vi "Meandr_FIFO_target.vi"() -> ()   [LabVIEW 2018]
uses:
  <vilib>/Platform/TimedLoop/XDataNode/timing_clust.ctl
  <vilib>/Platform/TimedLoop/XDataNode/nitl_modes.ctl
  <vilib>/Platform/TimedLoop/XDataNode/wakeup.ctl
  <vilib>/rvi/Emulation/niFpgaGetClockAttributes.vi
  <vilib>/rvi/Emulation/niFpgaSctlEmulationGetInTimedLoop.vi
  <vilib>/rvi/Emulation/niFpgaEmulationReportErrorSimple.vi
  <vilib>/rvi/eio/common/nirviEmuTemplateMethod_errors.vi
  <vilib>/rvi/Emulation/niFpgaCriticalErrorInLSC.vi
  <vilib>/rvi/Emulation/niFpgaProcessEmulError.vi
  <vilib>/rvi/interface/RandomDataEmulation/niFpgaRandomDataHandleErrors.vi
  <vilib>/eio/EIONode/EIONode.xnode
  <vilib>/Platform/TimedLoop/XDataNode/XDataNode.xnode
  <vilib>/rvi/DataTransferAndStorage/Container/XNode/niFpgaContainer.xnode
  <vilib>/rvi/interface/RandomDataEmulation/nirviRandomDataFpgaReadWriteTemplate.vi
  <vilib>/Platform/TimedLoop/XDataNode/XDNodeRunTimeDep.lvlib
panel:
  in  "stop 2":bool
  in  "Push?":bool
  in  "Source Freq":refnum<k21>="100 MHz Clock"
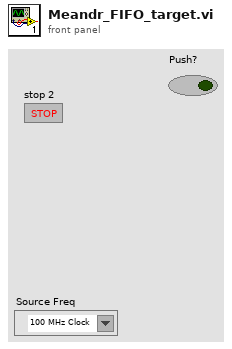
[diagram p1: front panel]
types:
  T1 = typedef "XDNodeRunTimeDep.lvlib/timing_clust.ctl" = cluster{"Expected End [f-1]":u64, "Actual End [f-1]":u64, "Finished Late? [f-1]":bool, "Expected End [i-1]":u64, "Actual End [i-1]":u64, "Finished Late? [i-1]":bool, "Expected Start [i]":u64, "Actual Start [i]":u64, "Expected Start [f]":u64, "Actual Start [f]":u64, "Source Name":string, "Structure Name":string, "Period":i64, "Deadline":i64, "Offset":i64, "Start":i64, "Priority":i32, "Timeout":i32, "Mode":T2, "Wakeup Reason":T3, "Error":errorcluster, "Source Type":string, "Secondary Source Type":string, "Global End Time":u64, "Global Start Time":u64, "Frame Duration":u64, "Iteration Duration":u64, "Assigned CPU":i32, "I/O Scan Engine Mode":u32}
  T2 = typedef "XDNodeRunTimeDep.lvlib/nitl_modes.ctl" = enum32{"No Change", "Process missed periods, maintain original phase", "Discard missed periods, maintain original phase", "Process missed periods, ignore original phase", "Discard missed periods, ignore original phase"}
  T3 = typedef "XDNodeRunTimeDep.lvlib/wakeup.ctl" = enum32{"Normal", "Aborted", "Asynchronous wakeup", "Timing source error", "Timed loop error", "Timeout"}
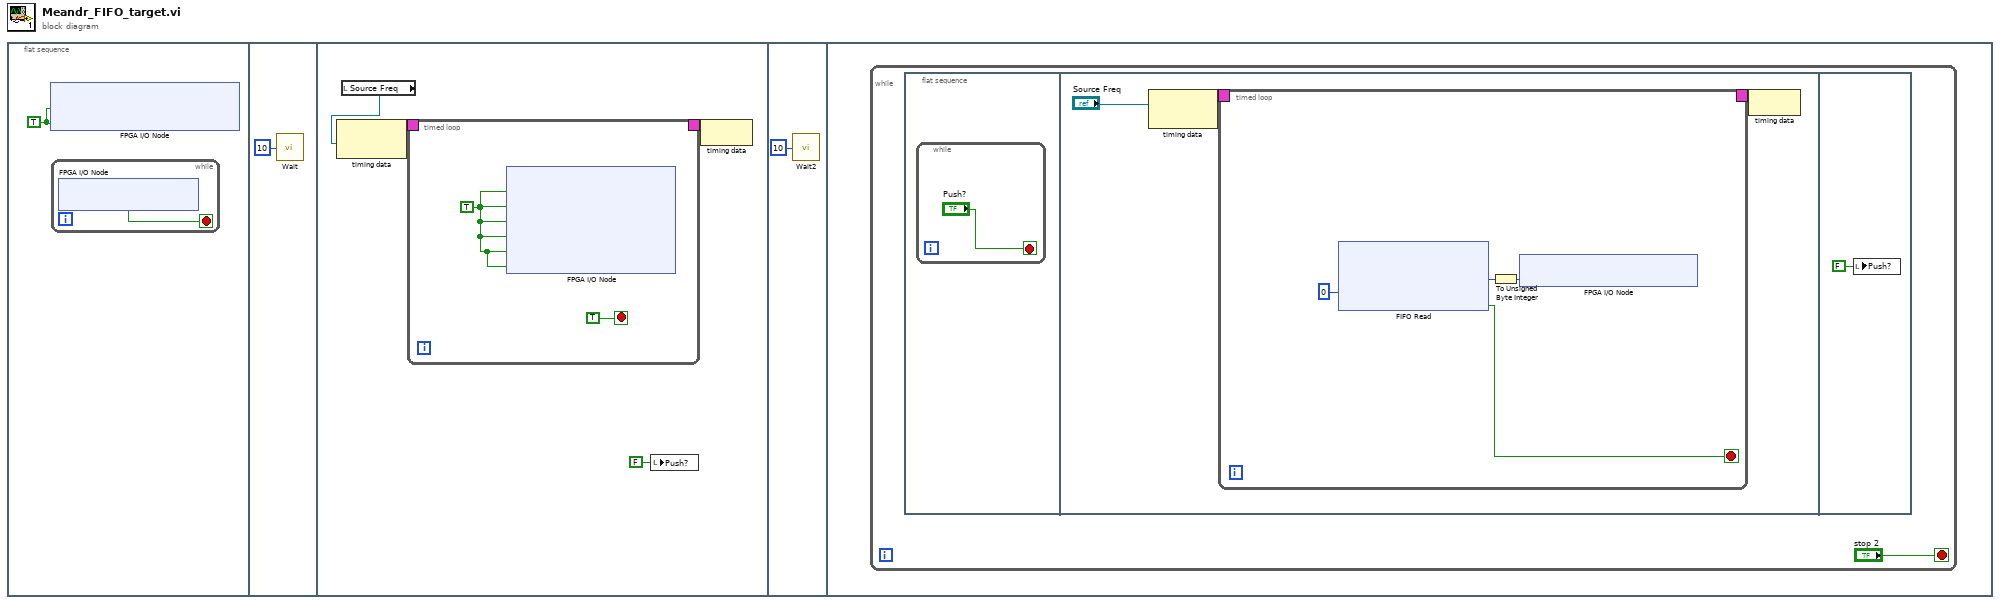
[diagram p0: block diagram]
diagram:
  n1 = flat-sequence {
    frame #0 {
      w1 = TRUE ("IO Module\\DDCB_Supply_Select")
      n2 = xnode "FPGA I/O Node"("IO Module\\DDCB_Supply_Select"=w1, "IO Module\\DDCA_Supply_Select"=w1) -> ()  [unwired: 2 in, 2 out]
      n3 = while {
        stop <- w2 stop-if-true
        n4 = xnode "FPGA I/O Node"() -> ("IO Module IO Enabled"=w2:bool)  [unwired: 1 in, 1 out]
      }
    }
    frame #1 {
      n5 = call "Wait"("Count(mSec)"=u8 10) -> ()  [unwired: 1 out]
    }
    frame #2 {
      n6 = local read "Source Freq"() -> (w5:refnum<k21>)
      n7 = node-c288(w5) -> (w7:T1)
      n8 = timed-loop {
        timing: w7 -> [_]
        timing-out: [_] -> w6
        stop <- TRUE stop-if-true
        w8 = TRUE
        n9 = xnode "FPGA I/O Node"("IO Module\\DDCA_Port0_WE"=w8, "IO Module\\DDCA_Port1_WE"=w8, "IO Module\\DDCA_Port2_WE"=w8, "IO Module\\DDCB_Port0_WE"=w8, "IO Module\\DDCB_Port1_WE"=w8, "IO Module\\DDCB_Port2_WE"=w8) -> ()  [unwired: 6 in, 6 out]
      }
      n10 = local write "Push?"(FALSE ("Push?")) -> ()
      n11 = node-c288(w6) -> ()
    }
    frame #3 {
      n12 = call "Wait2"("Count(mSec)"=u8 10) -> ()  [unwired: 1 out]
    }
    frame #4 {
      n13 = while {
        stop <- "stop 2" stop-if-true
        n14 = flat-sequence {
          frame #0 {
            n15 = while {
              stop <- "Push?" stop-if-true
            }
          }
          frame #1 {
            n16 = node-c288("Source Freq") -> (w21:T1)
            n17 = timed-loop {
              timing: w21 -> [_]
              timing-out: [_] -> w20
              stop <- w22 stop-if-true
              n18 = xnode ("FIFO Read")("Timeout"=0) -> ("Element"=w24:u8, "Timed Out?"=w22:bool)  [unwired: 1 in, 1 out]
              n19 = To Unsigned Byte Integer(number=w24) -> (unsigned 8bit integer=w25:u8)
              n20 = xnode "FPGA I/O Node"("IO Module\\DDCA_Port0_Write"=w25) -> ()  [unwired: 1 in, 1 out]
            }
            n21 = node-c288(w20) -> ()
          }
          frame #2 {
            n22 = local write "Push?"(FALSE ("Push?")) -> ()
          }
        }
      }
    }
  }
